vi "NeuronID_UDP_send_v002.vi"(2 "error in (no error)":errorcluster, 3 "Time":dbl(slide) scale=0.0..10.0, 5 "UDP Network Connection in":refnum<k16>) -> (0 "error out":errorcluster, 1 "UDP Network Connection out":refnum<k16>)   [LabVIEW 2019]
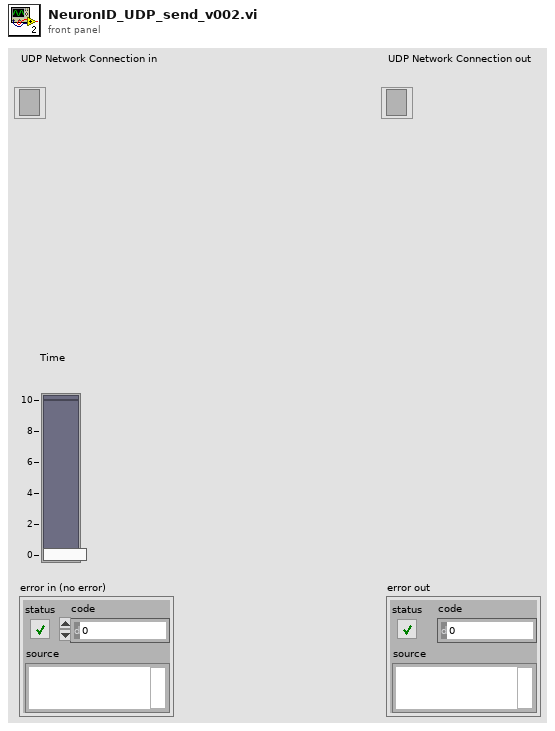
[diagram p1: front panel]
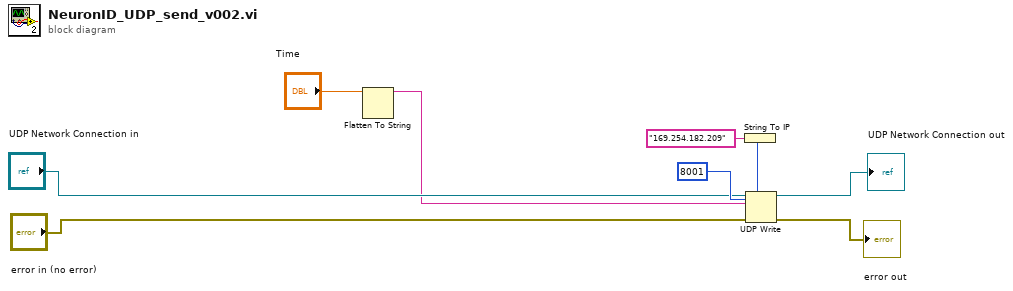
[diagram p0: block diagram]
diagram:
  n1 = Flatten To String(anything="Time") -> (data string=w1:string)  [unwired: 3 in, 2 out]
  n2 = String To IP(1:"169.254.182.209" ("name")) -> (0:w9:u32)
  n3 = UDP Write(address=w9, port or service name=u16 8001, connection ID="UDP Network Connection in", data in=w1, 8:"error in (no error)") -> (error out=→"error out":errorcluster, 3:→"UDP Network Connection out":refnum<k16>)  [unwired: 1 in]
